vi "Configure User Interface.vi"(6 "Beeper (F: Off)":bool, 7 "Lock-Out (F: Off)":bool, 8 "error in (no error)":errorcluster, 9 "Lock-Out Code (123)":i32=123 min=0 max=999 step=1, 10 "Remote Interface Mode (0: Local)":u16(ring) items=["Local", "Remote", "Remote w/ Lockout"], 11 "VISA resource name":refnum<visa-resource-name>) -> (0 "error out":errorcluster, 3 "VISA resource name out":refnum<visa-resource-name>)   [LabVIEW 2015, in "Lake Shore 372.lvlib"]
doc: "Configures various user interface settings. Parameters configured are;\nRemote interface mode, Keypad lock out, Audible beeper status."
uses:
  <instrlib>/Lake Shore 372/Lake Shore 372.lvlib
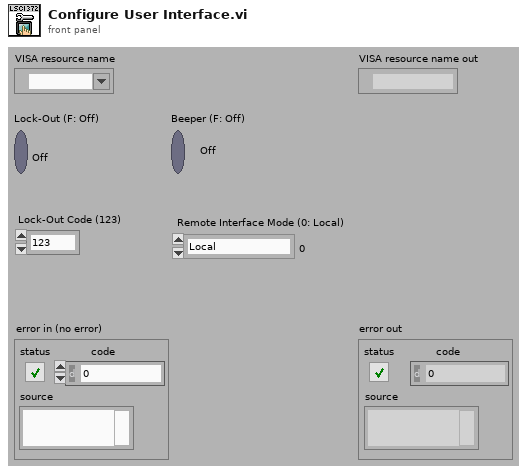
[diagram p1: front panel]
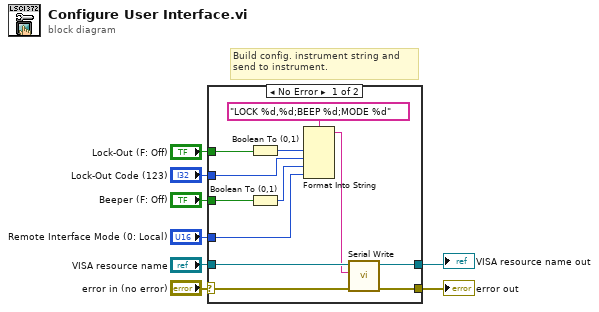
[diagram p0: block diagram]
diagram:
  # "Build config. instrument string and\nsend to instrument."
  n1 = case shown="No Error" "error in (no error)" {
    selector: "error in (no error)" -> [w9 w22]
    tunnel: "Lock-Out (F: Off)" -> [w20 _]
    tunnel: "Beeper (F: Off)" -> [w19 _]
    tunnel: "VISA resource name" -> [w18 w21]
    tunnel: [w17 w22] -> w5
    tunnel: [w16 w21] -> w4
    tunnel: "Lock-Out Code (123)" -> [w13 _]
    tunnel: "Remote Interface Mode (0: Local)" -> [w11 _]
    frame No Error {
      n2 = Boolean To (0,1)(Boolean=w20) -> (0, 1=w14:i16)
      n3 = Boolean To (0,1)(Boolean=w19) -> (0, 1=w12:i16)
      n4 = Format Into String(format string="LOCK %d,%d;BEEP %d;MODE %d", w14, w13, w12, w11) -> (resulting string=w10:string)  [unwired: 2 in, 1 out]
      n5 = call <instrlib>:"Serial Write.vi"("error in (no error)"=w9, "Write Buffer (\"\")"=w10, "VISA resource name"=w18) -> ("error out"=w17:errorcluster, "VISA resource name out"=w16:refnum<visa-resource-name>)  [unwired: 6 in, 1 out]
    }
    frame Error {
    }
  }
  "error out" <- w5
  "VISA resource name out" <- w4
